vi "Test Follow Redirects.vi"() -> ()   [LabVIEW 2020]
uses:
  classes/Response Headers/Response Headers.lvclass
  classes/REST Client/REST Client.lvclass/REST Client.ctl
  classes/REST Client/REST Client.lvclass
panel:
  out "Status Code":u16
  out "Status String":string
  out "Response Headers":refnum<class "Response Headers.lvclass">
  out "error out":errorcluster
  out "Response body":string
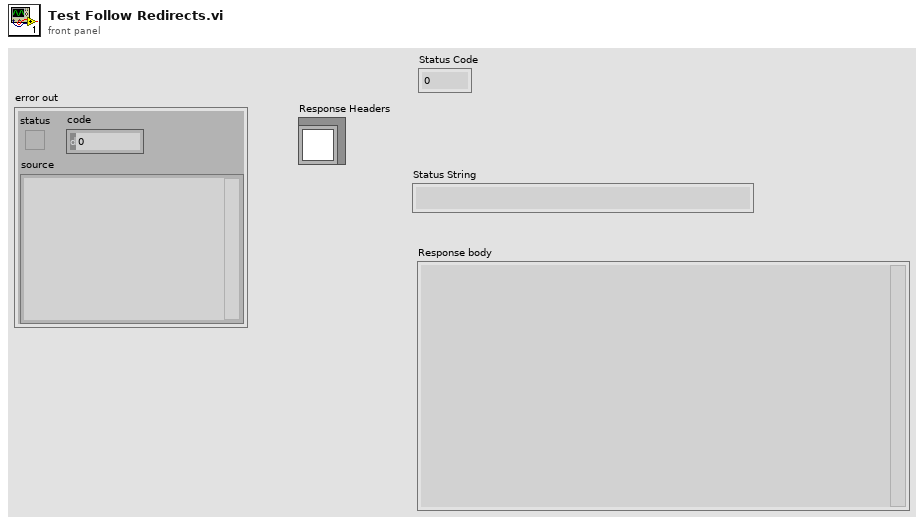
[diagram p1: front panel]
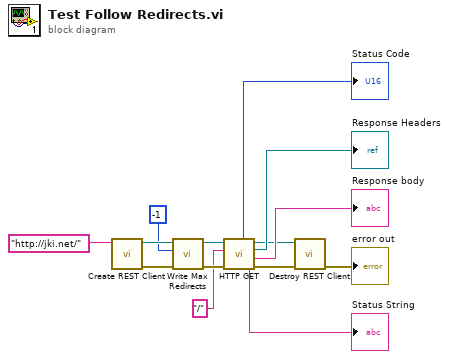
[diagram p0: block diagram]
diagram:
  n1 = call "Create REST Client.vi"("Base URL"="http://jki.net/") -> ("error out"=w8:errorcluster, "REST Client out"=w10:refnum<class "REST Client.lvclass">)  [unwired: 9 in]
  n2 = call "Write Max Redirects.vi"("error in (no error)"=w8, "max redirects (-1 = no limit)"=-1, "REST Client in"=w10) -> ("error out"=w7:errorcluster, "REST Client out"=w6:refnum<class "REST Client.lvclass">)  [unwired: 7 in]
  n3 = call-dynamic "HTTP GET.vi"("error in (no error)"=w7, "Path"="/", "REST Client in"=w6) -> ("error out"=w4:errorcluster, "Response body"=→"Response body":string, "Response Headers"=→"Response Headers":refnum<class "Response Headers.lvclass">, "REST Client out"=w5:refnum<class "REST Client.lvclass">, "Status String"=→"Status String":string, "Status Code"=→"Status Code":u16)  [unwired: 3 in]
  n4 = call-dynamic "Destroy REST Client.vi"("error in (no error)"=w4, "REST Client in"=w5) -> ("error out"=→"error out":errorcluster)  [unwired: 9 in]
